vi "Global calib.vi"() -> ()   [LabVIEW 2024]
panel:
  in  "calib":bool
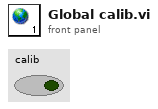
[diagram p1: front panel]
diagram:
